vi "Generate Random Material Design Color.vi"() -> (3 "Random colors":T1)   [LabVIEW 2020, in "Process Generation.lvlib" / "Process Generator.lvclass"]
uses:
  Process Generator.lvclass
  <vilib>/LabVIEW Icon API/API_Rectangle Colors.ctl
  <vilib>/LabVIEW Icon API/LabVIEW Icon API.lvlib
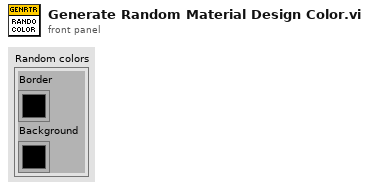
[diagram p1: front panel]
types:
  T1 = typedef "LabVIEW Icon API.lvlib/API_Rectangle Colors.ctl" = cluster{"Border":u32, "Background":u32}
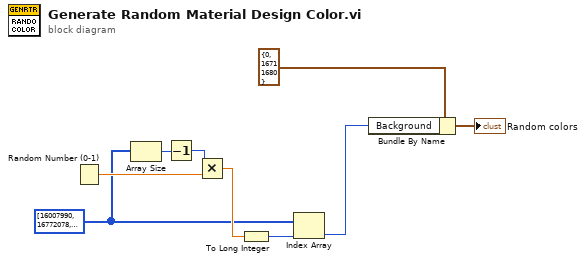
[diagram p0: block diagram]
diagram:
  w1 = u32[] [16007990, 16772078, 16764370, 15702682, 15037299, 15684432, 15022389, 13840175, 12986408, 12000284, 16747136, 16732754, 16717636, 13959168, 16573676, 16301008, 16027569, 15753874, 15483002, 15277667, 14162784, 12720219, 11342935, 8916559, 16744619, 16728193, 16056407, 12915042, 15984117, 14794471, 13538264, 12216520, 11225020, 10233776, 9315498, 8069026, 6953882, 4854924, 15368444, 14696699, 13959417, 11141375, 15591414, 13747433, 11771355, 9795021, 8280002, 6765239, 6174129, 5320104, 4532128, 3218322, 11766015, 8146431, 6627327, 6422762, 15264502, 12962537, 10463450, 7964363, 6056896, 4149685, 3754411, 3162015, 2635155, 1713022, 9215743, 5467646, 4020990, 3166206, 14938877, 12312315, 9489145, 6600182, 4367861, 2201331, 2001125, 1668818, 1402304, 870305, 8565247, 4492031, 2718207, 2712319, 14808574, 11789820, 8508666, 5227511, 2733814, 240116, 236517, 166097, 161725, 87963, 8444159, 4244735, 45311, 37354, 14743546, 11725810, 8445674, 5099745, 2541274, 48340, 44225, 38823, 33679, 24676, 8716287, 1638399, 58879, 47316, 14742257, 11722715, 8440772, 5093036, 2533018, 38536, 35195, 31083, 26972, 19776, 11010027, 6619098, 1960374, 49061, 15267305, 13166281, 10868391, 8505220, 6732650, 5025616, 4431943, 3706428, 3046706, 1793568, 12187338, 6942894, 58998, 51283, 15857897, 14478792, 12968357, 11457921, 10275941, 9159498, 8172354, 6856504, 5606191, 3369246, 13434768, 11730777, 7798531, 6610199, 16382951, 15791299, 15134364, 14477173, 13951319, 13491257, 12634675, 11514923, 10394916, 8550167, 16056193, 15662913, 13041408, 11463168, 16776679, 16775620, 16774557, 16773494, 16772696, 16771899, 16635957, 16498733, 16361509, 16088855, 16777101, 16776960, 16771584, 16766464, 16775393, 16772275, 16769154, 16766287, 16763432, 16761095, 16757504, 16752640, 16748288, 16740096, 16770431, 16766784, 16761856, 16755456, 16774112, 16769202, 16764032, 16758605, 16754470, 16750592, 16485376, 16088064, 15690752, 15094016, 16765312, 16755520, 16748800, 16739584, 16509415, 16764092, 16755601, 16747109, 16740419, 16733986, 16011550, 15092249, 14172949, 12531212, 16752256, 16739904, 16727296, 14494720, 15723497, 14142664, 12364452, 10586239, 9268835, 7951688, 7162945, 6111287, 5125166, 4073251, 16448250, 16119285, 15658734, 14737632, 12434877, 10395294, 7697781, 6381921, 4342338, 2171169, 15527921, 13621468, 11583173, 9479342, 7901340, 6323595, 5533306, 4545124, 3622735, 2503224] ("number")
  n1 = Random Number (0-1)() -> (number: 0 to 1=w6:dbl)
  n2 = Array Size(array=w1) -> (size(s)=w7:i32)
  n3 = Decrement(x=w7) -> (x-1=w2:i32)
  n4 = Multiply(x=w2, y=w6) -> (x*y=w5:dbl)
  n5 = To Long Integer(number=w5) -> (32bit integer=w4:i32)
  n6 = Index Array(array=w1, index=w4) -> (element=w3:u32)
  n7 = Bundle By Name(cluster=T1 {"Border"=0, "Background"=16711680} ("Rectangle colors (black, white)"), "Background"=w3) -> (→"Random colors":T1)
